vi "channeldata.vi"() -> ()   [LabVIEW 2019]
panel:
  out "Error Out":errorcluster
  in  "TDMS File":path=path "C:/Python/projects/nitdms/tests/tdms_files/channeldata.tdms"
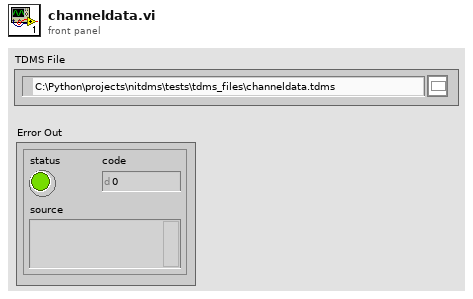
[diagram p1: front panel]
types:
  T1 = enum16{"open", "open or create", "create or replace", "create", "open (read-only)"}
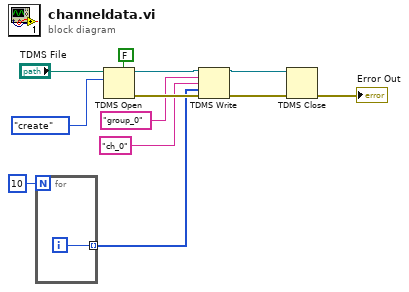
[diagram p0: block diagram]
diagram:
  n1 = for {
    N: 10 -> [_]
    tunnel: [w13] -> w1 mode=indexing
    i -> [w13]
  }
  n2 = TDMS Open(5:FALSE ("create index file? (T)"), 10:T1."create" ("operation (0:open)"), 11:"TDMS File") -> (0:w8:errorcluster, 3:w7:refnum<k34>)  [unwired: 4 in]
  n3 = TDMS Write(0:w7, 5:"group_0", 7:"ch_0", 9:w1, 11:w8) -> (4:w5:refnum<k34>, 15:w6:errorcluster)  [unwired: 1 in, 2 out]
  n4 = TDMS Close(8:w6, 11:w5) -> (0:→"Error Out":errorcluster)  [unwired: 1 out]
